vi "Typecast Queue to Refnum.vi"(11 "queue in":refnum<queue>) -> (3 "refnum out":refnum<k1>)   [LabVIEW 2017, in "NI_LVConfig.lvlib"]
uses:
  NI_LVConfig.lvlib
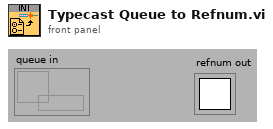
[diagram p1: front panel]
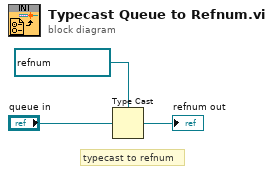
[diagram p0: block diagram]
diagram:
  w2 = refnum<k1> refnum items=["config data"] ("refnum out")
  # "typecast to refnum"
  n1 = Type Cast(type=w2, x="queue in") -> (*(type *) &x=→"refnum out":refnum<k1>)
